vi "SensorLoop.vi"   [LabVIEW 2018]
uses:
  <vilib>/Platform/TimedLoop/XDataNode/timing_clust.ctl
  <vilib>/Platform/TimedLoop/XDataNode/nitl_modes.ctl
  <vilib>/Platform/TimedLoop/XDataNode/wakeup.ctl
  <vilib>/Rock Robotics/Network Tables/NT Read Number.vi
  <vilib>/platform/TimedLoop/XDataNode/XDataNode.xnode
  <vilib>/Platform/TimedLoop/XDataNode/XDNodeRunTimeDep.lvlib
types:
  T1 = typedef "WPI_DigitalInputDevRef.ctl" = cluster{"DevStatus":errorcluster, "DIO Channel":T2}
  T2 = typedef "FPGA_DIOChannel.ctl" = enum8{"DIO 0", "DIO 1", "DIO 2", "DIO 3", "DIO 4", "DIO 5", "DIO 6", "DIO 7", "DIO 8", "DIO 9", "DIO MXP 0", "DIO MXP 1", "DIO MXP 2", "DIO MXP 3", "DIO MXP 4", "DIO MXP 5", "DIO MXP 6", "DIO MXP 7", "DIO MXP 8", "DIO MXP 9", "DIO MXP 10", "DIO MXP 11", "DIO MXP 12", "DIO MXP 13", "DIO MXP 14", "DIO MXP 15", "SPI Port CS1", "SPI Port CS2", "SPI Port CS3", "SPI Port MISO", "SPI Port MOSI", "Invalid"}
  T3 = typedef "WPI_EncoderDevRef.ctl" = cluster{"DevStatus":errorcluster, "EncoderIndex":T4, "CounterIndex":T5, "DistancePerCount":dbl, "Decoding Type":T6}
  T4 = typedef "FPGA_EncoderIdx.ctl" = enum8{"Enc 0", "Enc 1", "Enc 2", "Enc 3", "Enc 4", "Enc 5", "Enc 6", "Enc 7", "Invalid"}
  T5 = typedef "FPGA_CounterCtrSystemIndex.ctl" = enum8{"Ctr 0", "Ctr 1", "Ctr 2", "Ctr 3", "Ctr 4", "Ctr 5", "Ctr 6", "Ctr 7", "Invalid"}
  T6 = typedef "WPI_EncoderType.ctl" = enum16{"1x", "2x", "4x"}
  T7 = typedef "ImuDevRef.ctl" = cluster{"I2CDevRef":T8, "Valid Cal File?":bool}
  T8 = typedef "WPI_I2CDevRef.ctl" = cluster{"DevStatus":errorcluster, "Device Address":u8, "Handle":i32, "I2C Bus":T9}
  T9 = typedef "i2c_bus.ctl" = enum16{"I2C On-Board", "I2C MXP", "Invalid"}
  T10 = typedef "XDNodeRunTimeDep.lvlib/timing_clust.ctl" = cluster{"Expected End [f-1]":u64, "Actual End [f-1]":u64, "Finished Late? [f-1]":bool, "Expected End [i-1]":u64, "Actual End [i-1]":u64, "Finished Late? [i-1]":bool, "Expected Start [i]":u64, "Actual Start [i]":u64, "Expected Start [f]":u64, "Actual Start [f]":u64, "Source Name":string, "Structure Name":string, "Period":i64, "Deadline":i64, "Offset":i64, "Start":i64, "Priority":i32, "Timeout":i32, "Mode":T11, "Wakeup Reason":T12, "Error":errorcluster, "Source Type":string, "Secondary Source Type":string, "Global End Time":u64, "Global Start Time":u64, "Frame Duration":u64, "Iteration Duration":u64, "Assigned CPU":i32, "I/O Scan Engine Mode":u32}
  T11 = typedef "XDNodeRunTimeDep.lvlib/nitl_modes.ctl" = enum32{"No Change", "Process missed periods, maintain original phase", "Discard missed periods, maintain original phase", "Process missed periods, ignore original phase", "Discard missed periods, ignore original phase"}
  T12 = typedef "XDNodeRunTimeDep.lvlib/wakeup.ctl" = enum32{"Normal", "Aborted", "Asynchronous wakeup", "Timing source error", "Timed loop error", "Timeout"}
  T13 = cluster{"X Gyro":dbl, "Y Gyro":dbl, "Z Gyro":dbl, "X Rate":dbl, "Y Rate":dbl, "Z Rate":dbl}
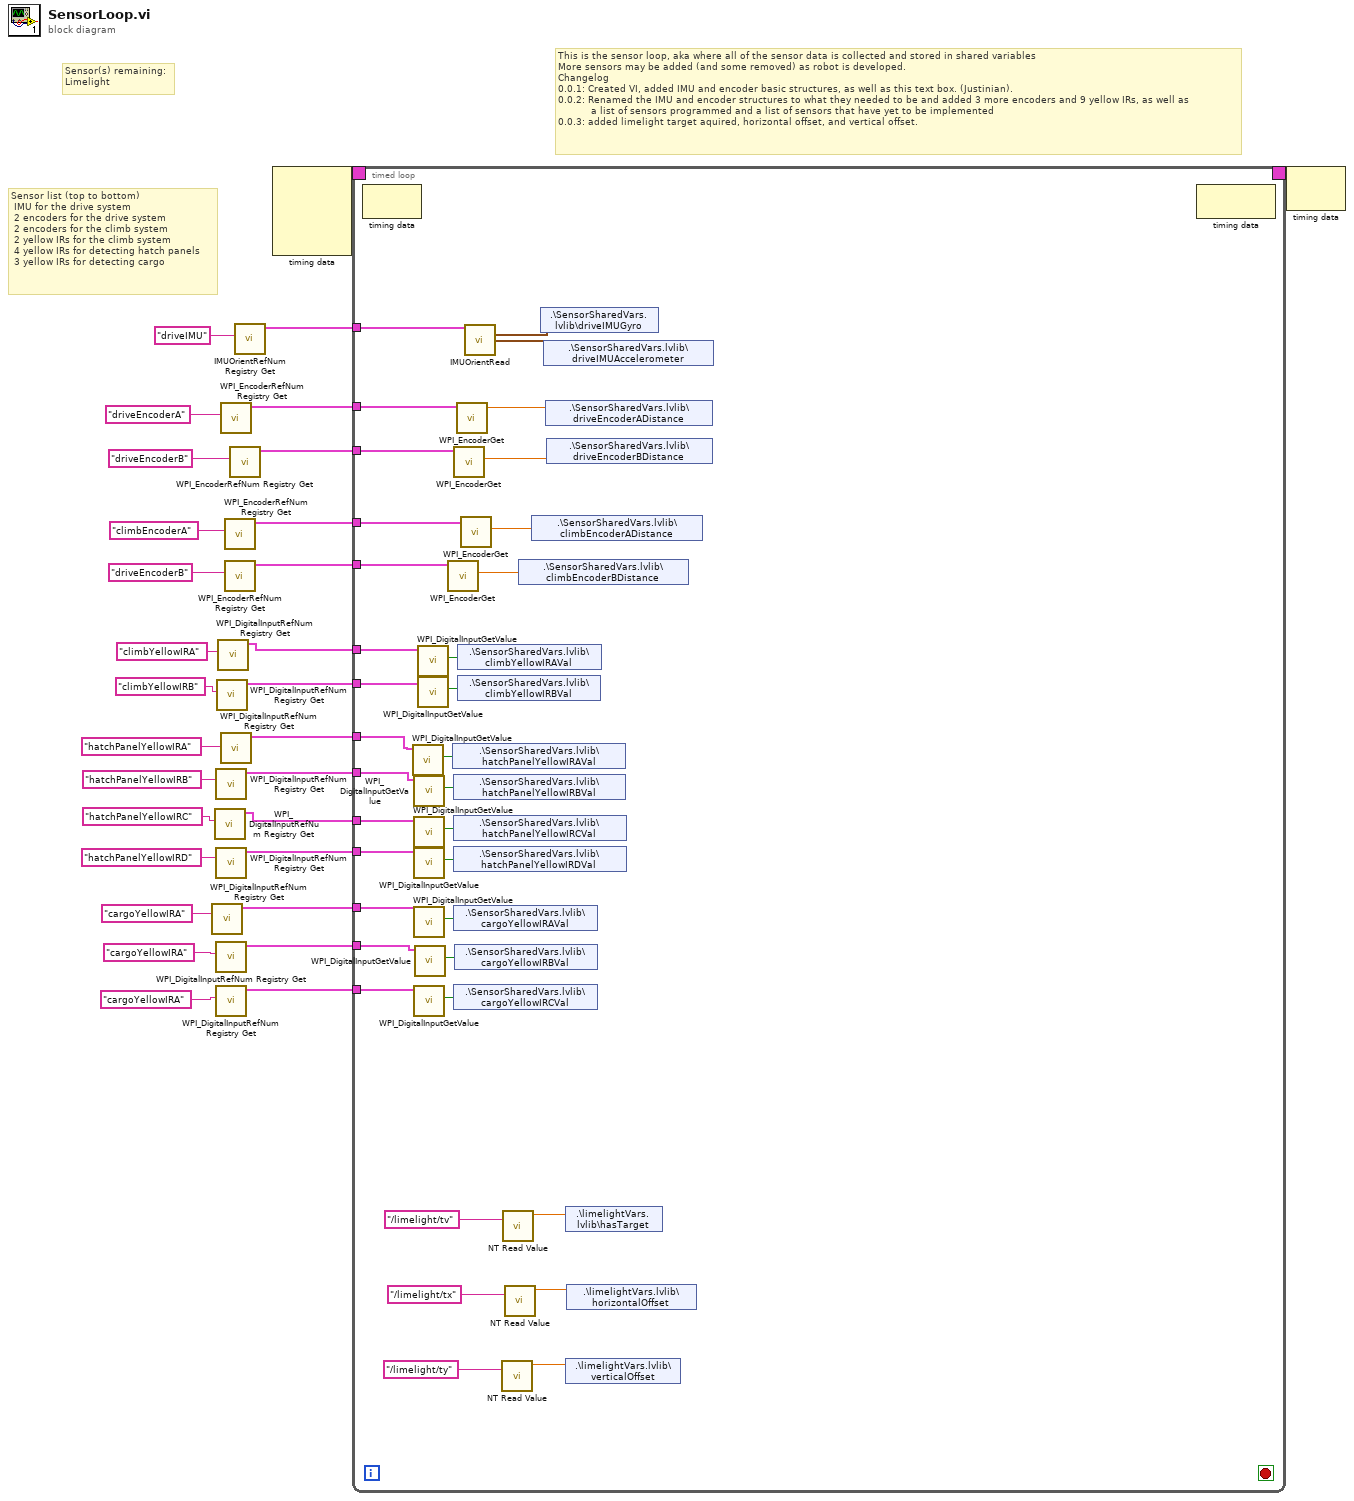
[diagram p0: block diagram]
diagram:
  # "Sensor(s) remaining:\nLimelight"
  # "Sensor list (top to bottom)\n IMU for the drive system\n 2 encoders for the drive system\n 2 encoders for the climb system\n 2 yellow IRs for the climb system\n 4 yellow IRs for detecting hatch panels\n 3 yellow IRs for detecting cargo"
  # "This is the sensor loop, aka where all of the sensor data is collected and stored in shared variables\nMore sensors may be added (and some removed) as robot is developed.\nChangelog\n0.0.1: Created VI, added IMU and encoder basic structures, as well as this text box. (Justinian).\n0.0.2: Renamed the IMU and encoder structures to what they needed to be and added 3 more encoders and 9 yellow IRs, as well as\n           a list of sensors programmed and a list of sensors that have yet to be implemented\n0.0.3: added limelight target aquired, horizontal offset, and vertical offset."
  n1 = call <vilib>:"WPI_DigitalInputRefNum Registry Get.vi"("refnum name"="cargoYellowIRA") -> ("DigitalInputDevRef"=w3:T1)  [unwired: 9 in, 1 out]
  n2 = call <vilib>:"WPI_DigitalInputRefNum Registry Get.vi"("refnum name"="hatchPanelYellowIRC") -> ("DigitalInputDevRef"=w5:T1)  [unwired: 9 in, 1 out]
  n3 = call <vilib>:"WPI_DigitalInputRefNum Registry Get.vi"("refnum name"="hatchPanelYellowIRB") -> ("DigitalInputDevRef"=w6:T1)  [unwired: 9 in, 1 out]
  n4 = call <vilib>:"WPI_DigitalInputRefNum Registry Get.vi"("refnum name"="hatchPanelYellowIRD") -> ("DigitalInputDevRef"=w4:T1)  [unwired: 9 in, 1 out]
  n5 = call <vilib>:"WPI_DigitalInputRefNum Registry Get.vi"("refnum name"="cargoYellowIRA") -> ("DigitalInputDevRef"=w2:T1)  [unwired: 9 in, 1 out]
  n6 = call <vilib>:"WPI_DigitalInputRefNum Registry Get.vi"("refnum name"="cargoYellowIRA") -> ("DigitalInputDevRef"=w1:T1)  [unwired: 9 in, 1 out]
  n7 = call <vilib>:"WPI_DigitalInputRefNum Registry Get.vi"("refnum name"="climbYellowIRB") -> ("DigitalInputDevRef"=w8:T1)  [unwired: 9 in, 1 out]
  n8 = call <vilib>:"WPI_DigitalInputRefNum Registry Get.vi"("refnum name"="climbYellowIRA") -> ("DigitalInputDevRef"=w9:T1)  [unwired: 9 in, 1 out]
  n9 = call <vilib>:"WPI_EncoderRefNum Registry Get.vi"("refnum name"="driveEncoderA") -> ("EncoderDevRef"=w28:T3)  [unwired: 9 in, 1 out]
  n10 = call <vilib>:"WPI_DigitalInputRefNum Registry Get.vi"("refnum name"="hatchPanelYellowIRA") -> ("DigitalInputDevRef"=w7:T1)  [unwired: 9 in, 1 out]
  n11 = call <vilib>:"WPI_EncoderRefNum Registry Get.vi"("refnum name"="climbEncoderA") -> ("EncoderDevRef"=w21:T3)  [unwired: 9 in, 1 out]
  n12 = call <vilib>:"WPI_EncoderRefNum Registry Get.vi"("refnum name"="driveEncoderB") -> ("EncoderDevRef"=w20:T3)  [unwired: 9 in, 1 out]
  n13 = call <vilib>:"WPI_EncoderRefNum Registry Get.vi"("refnum name"="driveEncoderB") -> ("EncoderDevRef"=w23:T3)  [unwired: 9 in, 1 out]
  n14 = call <userlib>:"IMUOrientRefNum Registry Get.vi"("refnum name"="driveIMU") -> ("IMUDevRef out"=w27:T7)  [unwired: 9 in, 1 out]
  n15 = node-c288() -> (w30:T10)  [unwired: 4 in]
  n16 = timed-loop {
    timing: w30 -> [_]
    timing-out: [_] -> w29
    tunnel: w28 -> [w64]
    tunnel: w27 -> [w63]
    tunnel: w23 -> [w60]
    tunnel: w21 -> [w58]
    tunnel: w20 -> [w57]
    tunnel: w9 -> [w54]
    tunnel: w8 -> [w53]
    tunnel: w7 -> [w52]
    tunnel: w6 -> [w51]
    tunnel: w5 -> [w50]
    tunnel: w4 -> [w49]
    tunnel: w3 -> [w48]
    tunnel: w2 -> [w47]
    tunnel: w1 -> [w46]
    stop <- _ stop-if-true
    n17 = node-c288() -> ()  [unwired: 1 in, 1 out]
    n18 = call <vilib>:"WPI_DigitalInputGetValue.vi"("DigitalInputDevRef"=w52) -> ("Value"=w43:bool)  [unwired: 8 in, 2 out]
    n19 = call <vilib>:"WPI_DigitalInputGetValue.vi"("DigitalInputDevRef"=w51) -> ("Value"=w42:bool)  [unwired: 8 in, 2 out]
    n20 = call <vilib>:"WPI_DigitalInputGetValue.vi"("DigitalInputDevRef"=w50) -> ("Value"=w41:bool)  [unwired: 8 in, 2 out]
    n21 = call <vilib>:"WPI_DigitalInputGetValue.vi"("DigitalInputDevRef"=w49) -> ("Value"=w40:bool)  [unwired: 8 in, 2 out]
    n22 = call <vilib>:"WPI_DigitalInputGetValue.vi"("DigitalInputDevRef"=w48) -> ("Value"=w39:bool)  [unwired: 8 in, 2 out]
    n23 = call <vilib>:"WPI_DigitalInputGetValue.vi"("DigitalInputDevRef"=w46) -> ("Value"=w37:bool)  [unwired: 8 in, 2 out]
    n24 = call <vilib>:"WPI_DigitalInputGetValue.vi"("DigitalInputDevRef"=w47) -> ("Value"=w38:bool)  [unwired: 8 in, 2 out]
    n25 = call <vilib>:"WPI_DigitalInputGetValue.vi"("DigitalInputDevRef"=w54) -> ("Value"=w45:bool)  [unwired: 8 in, 2 out]
    n26 = call <vilib>:"WPI_DigitalInputGetValue.vi"("DigitalInputDevRef"=w53) -> ("Value"=w44:bool)  [unwired: 8 in, 2 out]
    n27 = call <vilib>:"WPI_EncoderGet.vi"("EncoderDevRef"=w57) -> ("Distance"=w55:dbl)  [unwired: 5 in, 5 out]
    n28 = shared-variable ".\\SensorSharedVars.lvlib\\hatchPanelYellowIRAVal"(w43) -> ()  [unwired: 1 in, 1 out]
    n29 = call <vilib>:"WPI_EncoderGet.vi"("EncoderDevRef"=w60) -> ("Distance"=w59:dbl)  [unwired: 5 in, 5 out]
    n30 = shared-variable ".\\SensorSharedVars.lvlib\\hatchPanelYellowIRBVal"(w42) -> ()  [unwired: 1 in, 1 out]
    n31 = shared-variable ".\\SensorSharedVars.lvlib\\hatchPanelYellowIRCVal"(w41) -> ()  [unwired: 1 in, 1 out]
    n32 = shared-variable ".\\SensorSharedVars.lvlib\\hatchPanelYellowIRDVal"(w40) -> ()  [unwired: 1 in, 1 out]
    n33 = shared-variable ".\\SensorSharedVars.lvlib\\cargoYellowIRAVal"(w39) -> ()  [unwired: 1 in, 1 out]
    n34 = shared-variable ".\\SensorSharedVars.lvlib\\cargoYellowIRCVal"(w37) -> ()  [unwired: 1 in, 1 out]
    n35 = shared-variable ".\\SensorSharedVars.lvlib\\cargoYellowIRBVal"(w38) -> ()  [unwired: 1 in, 1 out]
    n36 = call <vilib>:"WPI_EncoderGet.vi"("EncoderDevRef"=w64) -> ("Distance"=w65:dbl)  [unwired: 5 in, 5 out]
    n37 = shared-variable ".\\SensorSharedVars.lvlib\\climbYellowIRAVal"(w45) -> ()  [unwired: 1 in, 1 out]
    n38 = shared-variable ".\\SensorSharedVars.lvlib\\climbYellowIRBVal"(w44) -> ()  [unwired: 1 in, 1 out]
    n39 = call <vilib>:"WPI_EncoderGet.vi"("EncoderDevRef"=w58) -> ("Distance"=w56:dbl)  [unwired: 5 in, 5 out]
    n40 = call <userlib>:"IMUOrientRead.vi"("IMU Dev Ref"=w63) -> ("Gyro X,Y,Z"=w61:T13, "Acc X,Y,Z"=w62:cluster{"X Acc":dbl, "Y Acc":dbl, "Z Acc":dbl})  [unwired: 7 in, 6 out]
    n41 = call-poly <vilib>:"NT Read Value.vi"("Name"="/limelight/ty") -> ("Numeric"=w31:dbl)  [unwired: 9 in, 1 out]
    n42 = call-poly <vilib>:"NT Read Value.vi"("Name"="/limelight/tv") -> ("Numeric"=w33:dbl)  [unwired: 9 in, 1 out]
    n43 = call-poly <vilib>:"NT Read Value.vi"("Name"="/limelight/tx") -> ("Numeric"=w32:dbl)  [unwired: 9 in, 1 out]
    n44 = shared-variable ".\\SensorSharedVars.lvlib\\climbEncoderBDistance"(w55) -> ()  [unwired: 1 in, 1 out]
    n45 = shared-variable ".\\SensorSharedVars.lvlib\\climbEncoderADistance"(w56) -> ()  [unwired: 1 in, 1 out]
    n46 = shared-variable ".\\SensorSharedVars.lvlib\\driveIMUGyro"(w61) -> ()  [unwired: 1 in, 1 out]
    n47 = shared-variable ".\\SensorSharedVars.lvlib\\driveIMUAccelerometer"(w62) -> ()  [unwired: 1 in, 1 out]
    n48 = shared-variable ".\\SensorSharedVars.lvlib\\driveEncoderADistance"(w65) -> ()  [unwired: 1 in, 1 out]
    n49 = shared-variable ".\\SensorSharedVars.lvlib\\driveEncoderBDistance"(w59) -> ()  [unwired: 1 in, 1 out]
    n50 = shared-variable ".\\limelightVars.lvlib\\hasTarget"(w33) -> ()  [unwired: 1 in, 1 out]
    n51 = shared-variable ".\\limelightVars.lvlib\\verticalOffset"(w31) -> ()  [unwired: 1 in, 1 out]
    n52 = shared-variable ".\\limelightVars.lvlib\\horizontalOffset"(w32) -> ()  [unwired: 1 in, 1 out]
    n53 = node-c288() -> ()  [unwired: 1 in, 1 out]
  }
  n54 = node-c288(w29) -> ()  [unwired: 1 out]
